vi "Graph.vi"(6 "Ring size (points) (1024)":u32=1024, 8 "error in (no error)":errorcluster, 9 "Store Ring? (f)":bool, 10 "Store History? (f)":bool, 11 "Collection in":refnum<class "Collection.lvclass">) -> (0 "error out":errorcluster, 1 "Ring Buffers":T5, 2 "History Buffers":T5, 3 "Collection out":refnum<class "Collection.lvclass">, 5 "Data Points":T1)   [LabVIEW 2023, in "Collection.lvclass"]
doc: "(Dynamic) Take a data point, then append it to an internal history buffer. Return the history buffer as a waveform array configured for graphing."
uses:
  Collection.lvclass
  Readable/TX Graph.ctl
  Readable/Data Points.ctl
  Readable/Data Point.ctl
  Readable/Time.ctl
  Readable/X.ctl
  Collection.lvclass/Collection.ctl
  Readable/Readable.lvclass
panel:
  # "Generate a waveform array for graphing."
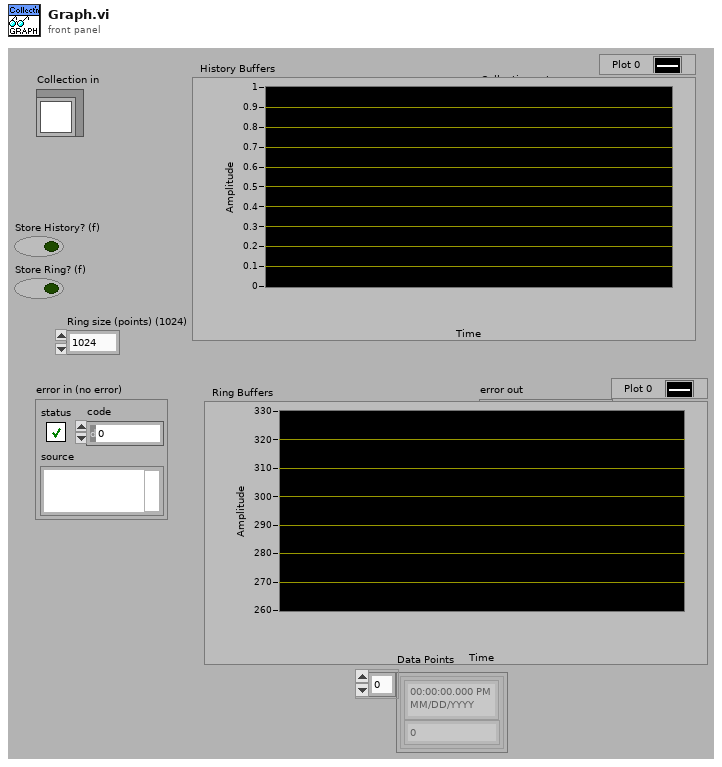
[diagram p1: front panel]
types:
  T1 = typedef "Readable.lvclass/Data Points.ctl" = T2[]
  T2 = typedef "Readable.lvclass/Data Point.ctl" = cluster{"t":T3, "x":T4}
  T3 = typedef "Readable.lvclass/Time.ctl" = timestamp
  T4 = typedef "Readable.lvclass/X.ctl" = dbl
  T5 = typedef "Readable.lvclass/TX Graph.ctl" = cluster{"Data Points":cluster{"t":timestamp, "x":dbl}[]}[]
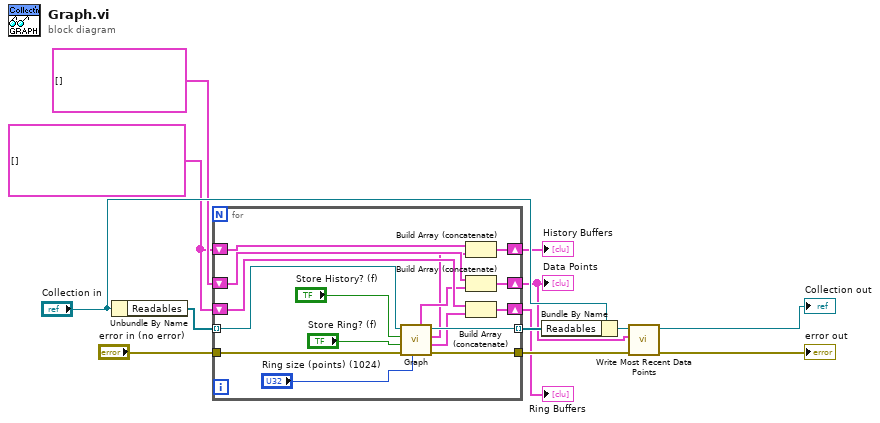
[diagram p0: block diagram]
diagram:
  w4 = T5 [] ("History Buffers")
  n1 = Unbundle By Name("Collection in") -> ("Readables"=w13:refnum<class "Readable.lvclass">[])
  n2 = for {
    tunnel: w13 -> [w23] mode=indexing
    tunnel: [w17] -> w11 mode=indexing
    tunnel: [w14] -> w9
    tunnel: "error in (no error)" -> [w20]
    shift-right: [w28] -> w1
    shift-left: T1 [] ("Data Points") -> [w29]
    shift-right: [w24] -> w2
    shift-left: w4 -> [w26]
    shift-right: [w25] -> w3
    shift-left: w4 -> [w27]
    n3 = call-dynamic "Graph.vi"("Ring size (points) (1024)"="Ring size (points) (1024)", "error in (no error)"=w20, "Store Ring? (f)"="Store Ring? (f)", "Store History? (f)"="Store History? (f)", "Readable in"=w23) -> ("error out"=w14:errorcluster, "Ring Buffers"=w15:T5, "History Buffers"=w16:T5, "Readable out"=w17:refnum<class "Readable.lvclass">, "Data Points"=w18:T1)  [unwired: 2 in]
    n4 = Build Array (concatenate)(w26, w16) -> (w24:T5)
    n5 = Build Array (concatenate)(w29, w18) -> (w28:T1)
    n6 = Build Array (concatenate)(w27, w15) -> (w25:T5)
  }
  "Ring Buffers" <- w3
  "History Buffers" <- w2
  "Data Points" <- w1
  n7 = Bundle By Name(cluster="Collection in", "Readables"=w11) -> (w10:refnum<class "Collection.lvclass">)
  n8 = call-dynamic "Write Most Recent Data Points.vi"("error in (no error)"=w9, "Data Points"=w1, "Readable in"=w10) -> ("error out"=→"error out":errorcluster, "Readable out"=→"Collection out":refnum<class "Collection.lvclass">)  [unwired: 7 in]
